vi "Begin.vi"(11 "Image Size":T1=enum."160x120") -> (0 "error out":errorcluster)   [LabVIEW 2012]
doc: "Called before other user functions, this VI is expected to open initial I/O refnums, load in file data, and do all program initialization. Notice that the <B>error out</B> terminal is simply used for data flow. Wiring it to other structures or subVIs ensures that this VI runs first."
uses:
  <vilib>/Rock Robotics/WPI/Camera/WPI_CameraImageSize.ctl
  <vilib>/Rock Robotics/WPI/Camera/WPI_CameraWhite Balance Values.ctl
  <vilib>/Rock Robotics/WPI/Camera/WPI_CameraExposure Values.ctl
  <vilib>/Rock Robotics/WPI/Camera/WPI_CameraFrameRate.ctl
  <vilib>/Rock Robotics/SystemInterfaces/DIO/FPGA_DIOPWMChannel.ctl
  <vilib>/Rock Robotics/WPI/Joystick/WPI_JoystickDeviceEnum.ctl
  <vilib>/Rock Robotics/SystemInterfaces/DIO/FPGA_DIOChannel.ctl
  <vilib>/Rock Robotics/WPI/Solenoid/WPI_SolenoidChannel.ctl
  <vilib>/Rock Robotics/SystemInterfaces/Typedef/FPGA_TypedefSolenoidModule.ctl
  <vilib>/Rock Robotics/SystemInterfaces/Typedef/FPGA_TypedefDigitalModule.ctl
  <vilib>/Rock Robotics/SystemInterfaces/DIO/FPGA_DIORelayChannel.ctl
  <vilib>/Rock Robotics/WPI/SafetyOutput/WPI_SafetyOutputConfigMenu.ctl
  <vilib>/Rock Robotics/WPI/MotorControl/WPI_MotorControlOpen Victor.vi
  <vilib>/Rock Robotics/WPI/Solenoid/WPI_SolenoidOpenSingle.vi
  <vilib>/Rock Robotics/WPI/MotorControl/WPI_MotorControlOpen Jaguar.vi
  Robot Global Data.vi
  <vilib>/Rock Robotics/WPI/RobotDrive/WPI_RobotDriveOpen4MotorWithJaguar.vi
  Autonomous Global Data.vi
  <vilib>/Rock Robotics/WPI/Compressor/WPI_CompressorGetSetRefNum.vi
  <vilib>/Rock Robotics/WPI/Encoder/WPI_EncoderType.ctl
  <vilib>/Rock Robotics/WPI/Counter/WPI_CounterDigitalInputToDigitalSource.vi
panel:
  out "1699-Autonomous.ini":string[][](array[string])=[["Autonomous Mode to run", "6"], ["Autonomous File No. to run (Mode 2 only)", "0"], ["Disance to Trave D1", "4.5"], ["Disance to Trave D2", "4.6"], ["Disance to Trave D3", "0"], ["Rate to tavel at R1", "-0.7"], ["Rate to tavel at R2", "-0.5"], ["Rate to tavel at R3", "0"], ["Key Shoot", "0"], ["Auto Type", "1"]]
  out "1699-preferences.ini":string[][](array[string])
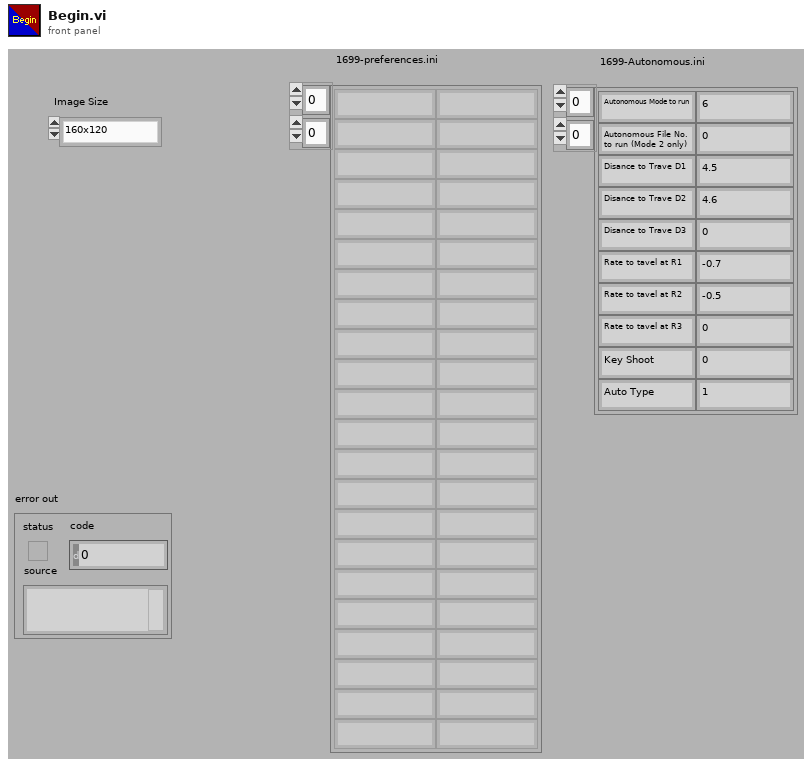
[diagram p1: front panel]
types:
  T1 = typedef "WPI_CameraImageSize.ctl" = enum16{"640x480", "320x240", "160x120"}
  T2 = typedef "WPI_SafetyOutputConfigMenu.ctl" = enum16{"Enable", "Disable"}
  T3 = typedef "FPGA_DIOChannel.ctl" = enum8{"DIO 1", "DIO 2", "DIO 3", "DIO 4", "DIO 5", "DIO 6", "DIO 7", "DIO 8", "DIO 9", "DIO 10", "DIO 11", "DIO 12", "DIO 13", "DIO 14", "Invalid"}
  T4 = typedef "FPGA_TypedefDigitalModule.ctl" = enum16{"Digital Module 1", "Digital Module 2"}
  T5 = typedef "FPGA_DIOPWMChannel.ctl" = enum8{"PWM 1", "PWM 2", "PWM 3", "PWM 4", "PWM 5", "PWM 6", "PWM 7", "PWM 8", "PWM 9", "PWM 10", "Invalid"}
  T6 = typedef "FPGA_DIORelayChannel.ctl" = enum8{"Relay 1", "Relay 2", "Relay 3", "Relay 4", "Relay 5", "Relay 6", "Relay 7", "Relay 8", "Invalid"}
  T7 = typedef "WPI_SolenoidChannel.ctl" = enum8{"Solenoid 1", "Solenoid 2", "Solenoid 3", "Solenoid 4", "Solenoid 5", "Solenoid 6", "Solenoid 7", "Solenoid 8", "Invalid"}
  T8 = typedef "FPGA_TypedefSolenoidModule.ctl" = enum16{"Solenoid Module 1", "Solenoid Module 2"}
  T9 = typedef "WPI_JoystickDeviceEnum.ctl" = enum16{"USB 1", "USB 2", "USB 3", "USB 4", "Kinect 1", "Kinect 2"}
  T10 = typedef "WPI_CameraFrameRate.ctl" = u32
  T11 = typedef "WPI_CameraExposure Values.ctl" = enum16{"Auto", "Flicker-free 50 Hz", "Flicker-free 60 Hz", "Hold current"}
  T12 = typedef "WPI_CameraWhite Balance Values.ctl" = enum16{"Auto", "Fixed indoor", "Fixed outdoor 1", "Fixed outdoor 2", "Fixed fluorescent 1", "Fixed fluorescent 2", "Hold current"}
  T13 = cluster{"[0]":dbl, "[1]":dbl, "[2]":dbl, "[3]":dbl, "[4]":dbl, "[5]":dbl, "[6]":dbl, "[7]":dbl, "[8]":dbl, "[9]":dbl, "[10]":dbl, "[11]":dbl, "[12]":dbl, "[13]":dbl, "[14]":dbl, "[15]":dbl, "[16]":dbl, "[17]":dbl, "[18]":dbl, "[19]":dbl}
  T14 = typedef "WPI_CameraDevRef.ctl" = cluster{"Camera Address":string, "CameraStatus":errorcluster, "Acquire Image Notifier":refnum<notifier>}
  T15 = typedef "WPI_RobotDriveDevRef.ctl" = cluster{"DevStatus":errorcluster, "Motors[]":T16[], "Square Inputs":bool, "Max Output":dbl, "Isochronous":bool}
  T16 = typedef "WPI_MotorControlDeviceRef.ctl" = cluster{"DeviceStatus":errorcluster, "Type":enum16{"PWM", "CAN"}, "PWM":cluster{"Digital Module":T4, "PWM Channel":T5, "DeadBand":T17}, "CAN":cluster{"Device Number":u8, "Control Mode":T18, "Semaphore":T19, "Max Vout":dbl}, "Invert":bool, "TransformRef":T20, "InvTransformRef":T20}
  T17 = typedef "WPI_PWMDeadband.ctl" = cluster{"Name":string, "maxPositivePwm":i32, "minPositivePwm":i32, "centerPwm":i32, "maxNegativePwm":i32, "minNegativePwm":i32, "angularRange":u16}
  T18 = typedef "WPI_CANJaguar_ControlMode.ctl" = enum8{"Percent VBus", "Current", "Speed", "Position", "Voltage"}
  T19 = typedef "Semaphore RefNum" = refnum<k1>
  T20 = typedef "WPI_PWMTransform_ConPane.ctl" = refnum<vi>
  T21 = typedef "WPI_EncoderType.ctl" = enum16{"1x", "2x", "4x"}
  T22 = typedef "WPI_DigitalInputDevRef.ctl" = cluster{"DevStatus":errorcluster, "DIO Channel":T3, "Digital Module":T4}
  T23 = typedef "FPGA_CounterEncoderSourceConvertionLVSourceType.ctl" = cluster{"DevStatus":errorcluster, "AnalogTriggerMode?":bool, "DigitalMode":cluster{"Digital Module":T4, "DIO Channel":T24}, "AnalogTriggerMode":cluster{"AnalogTriggerIndex":T25, "OutputType":T26}}
  T24 = typedef "FPGA_DIODigitalSourceChannel.ctl" = enum8{"DIO 1", "DIO 2", "DIO 3", "DIO 4", "DIO 5", "DIO 6", "DIO 7", "DIO 8", "DIO 9", "DIO 10", "DIO 11", "DIO 12", "DIO 13", "DIO 14", "Disabled"}
  T25 = typedef "FPGA_AnalogTriggerIndex.ctl" = enum8{"Trig 0", "Trig 1", "Trig 2", "Trig 3", "Trig 4", "Trig 5", "Trig 6", "Trig 7", "Invalid"}
  T26 = typedef "FPGA_AnalogTriggerOutType.ctl" = enum16{"InWindow", "TriggerState", "Rising", "Falling"}
  T27 = typedef "WPI_EncoderDevRef.ctl" = cluster{"DevStatus":errorcluster, "EncoderIndex":T28, "CounterIndex":T29, "DistancePerCount":dbl, "Decoding Type":T21}
  T28 = typedef "FPGA_EncoderIdx.ctl" = enum8{"Enc 0", "Enc 1", "Enc 2", "Enc 3", "Invalid"}
  T29 = typedef "FPGA_CounterCtrSystemIndex.ctl" = enum8{"Ctr 0", "Ctr 1", "Ctr 2", "Ctr 3", "Ctr 4", "Ctr 5", "Ctr 6", "Ctr 7", "Invalid"}
  T30 = typedef "WPI_JoystickDevRef.ctl" = cluster{"Device":T9}
  T31 = typedef "WPI_CompressorDevRef.ctl" = cluster{"DevStatus":errorcluster, "DigitalInputDevRef":T22, "RelayDevRef":T32}
  T32 = typedef "WPI_RelayDevRef.ctl" = cluster{"DevStatus":errorcluster, "Relay Channel":T6, "Digital Module":T4, "Relay Direction":T33}
  T33 = typedef "WPI_RelayDirection.ctl" = enum16{"Both directions", "Forward only", "Reverse only"}
  T34 = typedef "WPI_SolenoidDevRef.ctl" = cluster{"DevStatus":errorcluster, "Solenoid Module":T8, "Forward Solenoid Channel":T7, "Reverse Solenoid Channel":T7}
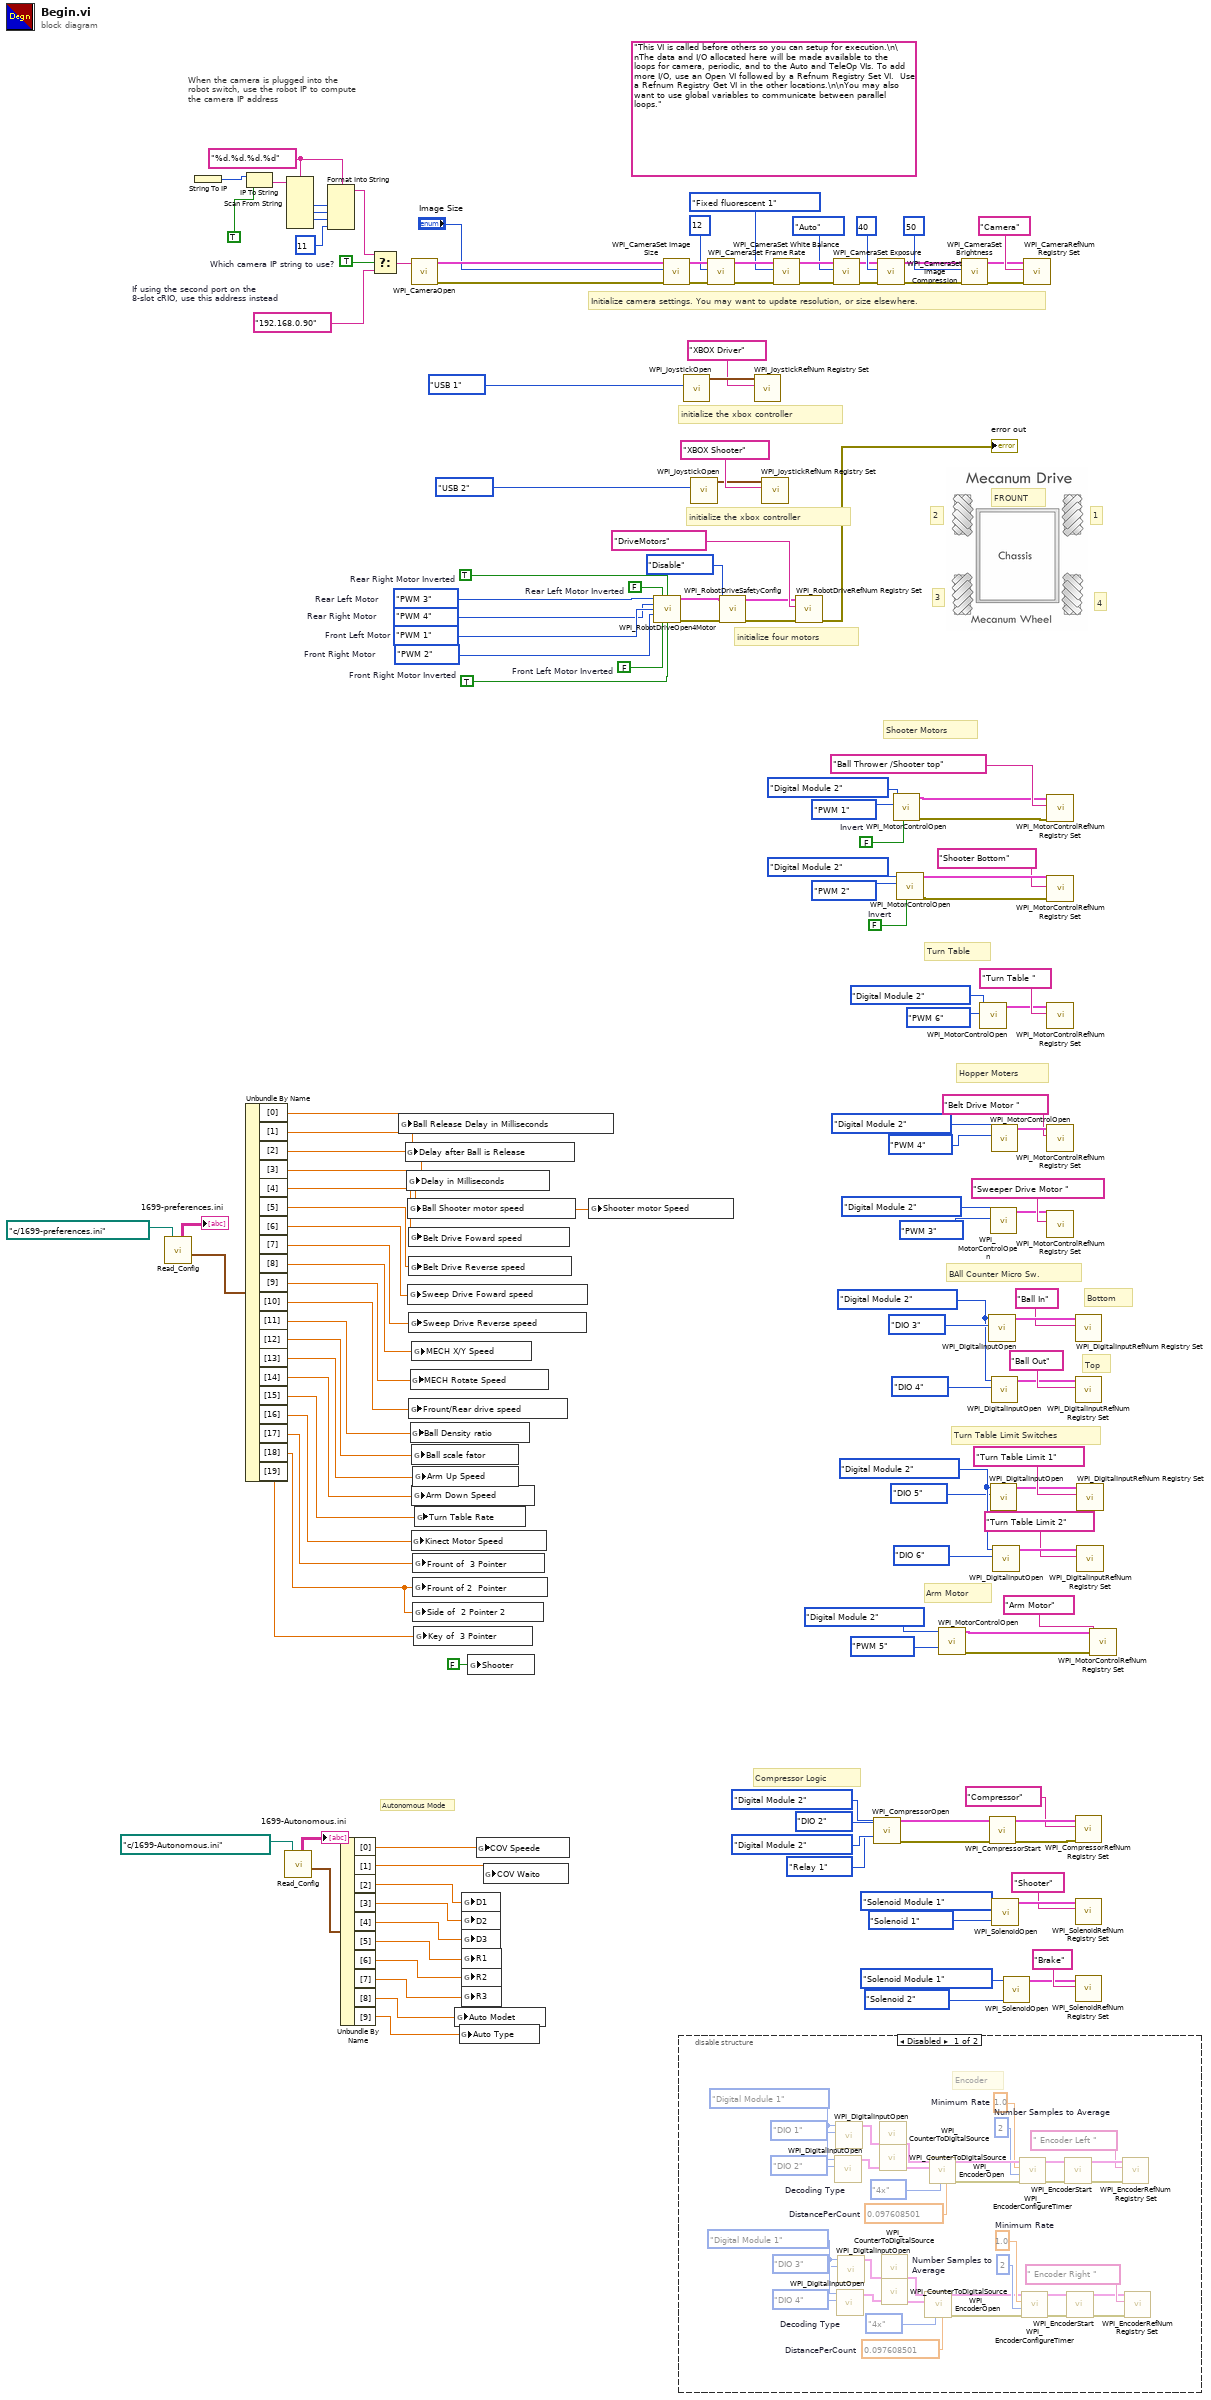
[diagram p0: block diagram]
diagram:
  w25 = FALSE  # Rear Left Motor Inverted
  w26 = FALSE  # Front Left Motor Inverted
  w36 = FPGA_TypedefDigitalModule."Digital Module 2" ("Digital Module (Module 1)")
  w43 = FALSE  # Invert
  w44 = FALSE  # Invert
  w94 = TRUE  # Front Right Motor Inverted
  w95 = TRUE  # Rear Right Motor Inverted
  w98 = FPGA_TypedefDigitalModule."Digital Module 2" ("Digital Module (Module 1)")
  w118 = FPGA_DIOPWMChannel."PWM 2"  # Front Right Motor
  w117 = FPGA_DIOPWMChannel."PWM 1"  # Front Left Motor
  w115 = FPGA_DIOPWMChannel."PWM 4"  # Rear Right Motor
  w114 = FPGA_DIOPWMChannel."PWM 3"  # Rear Left Motor
  w119 = TRUE  # Which camera IP string to use?
  w123 = "%d.%d.%d.%d" ("format string")
  (unwired) "This VI is called before others so you can setup for execution.\n\nThe data and I/O allocated here will be made available to the loops for camera, periodic, and to the Auto and TeleOp VIs. To add more I/O, use an Open VI followed by a Refnum Registry Set VI.  Use a Refnum Registry Get VI in the other locations.\n\nYou may also want to use global variables to communicate between parallel loops."
  w120 = "192.168.0.90"  # If using the second port on the 8-slot cRIO, use this address instead
  # "Autonomous Mode"
  # "FROUNT"
  # "Turn Table Limit Switches"
  # "Turn Table"
  # "Arm Motor"
  # "Top"
  # "Bottom"
  # "BAll Counter Micro Sw."
  # "Hopper Moters"
  # "Shooter Motors"
  # "Compressor Logic"
  # "initialize the xbox controller"
  # "1"
  # "4"
  # "3"
  # "2"
  # "initialize the xbox controller"
  # "initialize four motors"
  # "When the camera is plugged into the\nrobot switch, use the robot IP to compute\nthe camera IP address"
  # "Initialize camera settings. You may want to update resolution, or size elsewhere."
  n1 = call "Read_Config.vi"("configuration file path"=path "c:/1699-preferences.ini") -> ("PID Out"=w83:T13, "Array"=→"1699-preferences.ini":string[][])  [unwired: 2 in, 2 out]
  n2 = String To IP() -> (0:w130:u32)  [unwired: 1 in]
  n3 = Unbundle By Name(w83) -> ("[0]"=w93:dbl, "[1]"=w92:dbl, "[2]"=w91:dbl, "[3]"=w19:dbl, "[4]"=w90:dbl, "[5]"=w89:dbl, "[6]"=w88:dbl, "[7]"=w71:dbl, "[8]"=w70:dbl, "[9]"=w69:dbl, "[10]"=w68:dbl, "[11]"=w67:dbl, "[12]"=w66:dbl, "[13]"=w65:dbl, "[14]"=w64:dbl, "[15]"=w37:dbl, "[16]"=w29:dbl, "[17]"=w28:dbl, "[18]"=w20:dbl, "[19]"=w21:dbl)
  n4 = IP To String(1:TRUE ("dot notation? (F)"), 2:w130) -> (0:w128:string)
  n5 = call "Read_Config.vi"("configuration file path"=path "c:/1699-Autonomous.ini") -> ("PID Out"=w11:T13, "Array"=→"1699-Autonomous.ini":string[][])  [unwired: 2 in, 2 out]
  n6 = Scan From String(format string=w123, input string=w128) -> (output 1=w127:i32, output 2=w126:i32, output 3=w125:i32)  [unwired: 7 in, 3 out]
  n7 = Format Into String(format string=w123, w127, w126, w125, 11 ("Compression")) -> (resulting string=w121:string)  [unwired: 2 in, 1 out]
  n8 = Unbundle By Name(w11) -> ("[0]"=w10:dbl, "[1]"=w9:dbl, "[2]"=w8:dbl, "[3]"=w7:dbl, "[4]"=w6:dbl, "[5]"=w5:dbl, "[6]"=w4:dbl, "[7]"=w1:dbl, "[8]"=w3:dbl, "[9]"=w2:dbl)
  n9 = Select(t=w121, s=w119, f=w120) -> (s? t:f=w122:string)
  n10 = global write "Robot Global Data.vi" "Ball Release Delay in Milliseconds"(w93) -> ()
  n11 = global write "Robot Global Data.vi" "Delay after Ball is Release"(w92) -> ()
  n12 = global write "Robot Global Data.vi" "Delay in Milliseconds"(w91) -> ()
  n13 = global write "Robot Global Data.vi" "Ball Shooter motor speed"(w19) -> ()
  n14 = global write "Robot Global Data.vi" "Sweep Drive Foward speed"(w88) -> ()
  n15 = global write "Robot Global Data.vi" "Belt Drive Foward speed"(w90) -> ()
  n16 = global write "Robot Global Data.vi" "Belt Drive Reverse speed"(w89) -> ()
  n17 = global write "Robot Global Data.vi" "Sweep Drive Reverse speed"(w71) -> ()
  n18 = global write "Robot Global Data.vi" "Frount/Rear drive speed"(w68) -> ()
  n19 = global write "Robot Global Data.vi" "MECH Rotate Speed"(w69) -> ()
  n20 = global write "Robot Global Data.vi" "Ball Density ratio"(w67) -> ()
  n21 = call <vilib>:"WPI_CameraOpen.vi"("Camera Address"=w122) -> ("error out"=w142:errorcluster, "CameraDevRef"=w143:T14)  [unwired: 1 in, 8 out]
  n22 = global write "Robot Global Data.vi" "Kinect Motor Speed"(w29) -> ()
  n23 = global write "Robot Global Data.vi" "MECH X/Y Speed"(w70) -> ()
  n24 = global write "Robot Global Data.vi" "Ball scale fator"(w66) -> ()
  n25 = global write "Robot Global Data.vi" "Arm Down Speed"(w64) -> ()
  n26 = global write "Robot Global Data.vi" "Arm Up Speed"(w65) -> ()
  n27 = global write "Robot Global Data.vi" "Frount of  3 Pointer"(w28) -> ()
  n28 = global write "Robot Global Data.vi" "Frount of 2  Pointer"(w20) -> ()
  n29 = global write "Robot Global Data.vi" "Side of  2 Pointer 2"(w20) -> ()
  n30 = global write "Robot Global Data.vi" "Key of  3 Pointer"(w21) -> ()
  n31 = global write "Robot Global Data.vi" "Turn Table Rate"(w37) -> ()
  n32 = global write "Autonomous Global Data.vi" "Auto Modet"(w3) -> ()
  n33 = global write "Autonomous Global Data.vi" "Auto Type"(w2) -> ()
  n34 = global write "Autonomous Global Data.vi" "D1"(w8) -> ()
  n35 = global write "Autonomous Global Data.vi" "D2"(w7) -> ()
  n36 = global write "Autonomous Global Data.vi" "D3"(w6) -> ()
  n37 = global write "Autonomous Global Data.vi" "R1"(w5) -> ()
  n38 = global write "Autonomous Global Data.vi" "R2"(w4) -> ()
  n39 = global write "Autonomous Global Data.vi" "R3"(w1) -> ()
  n40 = global write "Robot Global Data.vi" "Shooter"(FALSE ("Shooter")) -> ()
  n41 = global write "Autonomous Global Data.vi" "COV Speede"(w10) -> ()
  n42 = global write "Autonomous Global Data.vi" "COV Waito"(w9) -> ()
  n43 = global write "Robot Global Data.vi" "Shooter motor Speed"(w19) -> ()
  n44 = call-poly <vilib>:"WPI_RobotDriveOpen4Motor.vi"("Rear Left Motor"=w114, "Rear Left Motor Inverted"=w25, "Rear Right Motor Inverted"=w95, "Rear Right Motor"=w115, "Front Left Motor"=w117, "Front Right Motor"=w118, "Front Left Motor Inverted"=w26, "Front Right Motor Inverted"=w94) -> ("RobotDriveDevRef"=w18:T15, "error out"=w15:errorcluster)  [unwired: 1 in, 5 out]
  n45 = call <vilib>:"WPI_CameraSet Image Size.vi"("error in (no error)"=w142, "Image Size"="Image Size", "CameraDevRef"=w143) -> ("error out"=w141:errorcluster, "CameraDevRef Out"=w144:T14)  [unwired: 7 out]
  n46 = disable-structure shown="Disabled" {
    frame Disabled {
      w169 = FPGA_TypedefDigitalModule."Digital Module 1" ("Digital Module (Module 1)")
      w162 = 0.097608501  # DistancePerCount
      w161 = WPI_EncoderType."4x"  # Decoding Type
      w160 = u8 2  # Number Samples to Average
      w159 = 1.0  # Minimum Rate
      w170 = FPGA_TypedefDigitalModule."Digital Module 1" ("Digital Module (Module 1)")
      w177 = 0.097608501  # DistancePerCount
      w178 = WPI_EncoderType."4x"  # Decoding Type
      w179 = u8 2  # Number Samples to Average
      w180 = 1.0  # Minimum Rate
      # "Encoder"
      n47 = call <vilib>:"WPI_DigitalInputOpen.vi"("DIO Channel"=FPGA_DIOChannel."DIO 2", "Digital Module (Module 1)"=w170) -> ("DigitalInputDevRef"=w174:T22)  [unwired: 8 in, 1 out]
      n48 = call <vilib>:"WPI_DigitalInputOpen.vi"("DIO Channel"=FPGA_DIOChannel."DIO 1", "Digital Module (Module 1)"=w170) -> ("DigitalInputDevRef"=w173:T22)  [unwired: 8 in, 1 out]
      n49 = call <vilib>:"WPI_DigitalInputOpen.vi"("DIO Channel"=FPGA_DIOChannel."DIO 4", "Digital Module (Module 1)"=w169) -> ("DigitalInputDevRef"=w165:T22)  [unwired: 8 in, 1 out]
      n50 = call <vilib>:"WPI_DigitalInputOpen.vi"("DIO Channel"=FPGA_DIOChannel."DIO 3", "Digital Module (Module 1)"=w169) -> ("DigitalInputDevRef"=w166:T22)  [unwired: 8 in, 1 out]
      n51 = call-poly <vilib>:"WPI_CounterToDigitalSource.vi"("DigitalInputDevRef"=w173) -> ("Digital Source"=w175:T23)  [unwired: 6 in]
      n52 = call-poly <vilib>:"WPI_CounterToDigitalSource.vi"("DigitalInputDevRef"=w174) -> ("Digital Source"=w176:T23)  [unwired: 6 in]
      n53 = call-poly <vilib>:"WPI_CounterToDigitalSource.vi"("DigitalInputDevRef"=w166) -> ("Digital Source"=w164:T23)  [unwired: 6 in]
      n54 = call-poly <vilib>:"WPI_CounterToDigitalSource.vi"("DigitalInputDevRef"=w165) -> ("Digital Source"=w163:T23)  [unwired: 6 in]
      n55 = call <vilib>:"WPI_EncoderOpen.vi"("DistancePerCount"=w162, "Decoding Type"=w161, "BSource"=w163, "ASource"=w164) -> ("error out"=w158:errorcluster, "EncoderDevRef"=w152:T27)  [unwired: 6 in]
      n56 = call <vilib>:"WPI_EncoderOpen.vi"("DistancePerCount"=w177, "Decoding Type"=w178, "BSource"=w176, "ASource"=w175) -> ("error out"=w181:errorcluster, "EncoderDevRef"=w187:T27)  [unwired: 6 in]
      n57 = call <vilib>:"WPI_EncoderConfigureTimer.vi"("error in (no error)"=w181, "Number Samples to Average"=w179, "Minimum Rate"=w180, "EncoderDevRef"=w187) -> ("error out"=w182:errorcluster, "EncoderDevRef"=w186:T27)  [unwired: 6 in]
      n58 = call <vilib>:"WPI_EncoderConfigureTimer.vi"("error in (no error)"=w158, "Number Samples to Average"=w160, "Minimum Rate"=w159, "EncoderDevRef"=w152) -> ("error out"=w157:errorcluster, "EncoderDevRef"=w153:T27)  [unwired: 6 in]
      n59 = call <vilib>:"WPI_EncoderStart.vi"("error in (no error)"=w182, "EncoderDevRef"=w186) -> ("error out"=w183:errorcluster, "EncoderDevRef"=w185:T27)  [unwired: 8 in]
      n60 = call <vilib>:"WPI_EncoderStart.vi"("error in (no error)"=w157, "EncoderDevRef"=w153) -> ("error out"=w156:errorcluster, "EncoderDevRef"=w154:T27)  [unwired: 8 in]
      n61 = call <vilib>:"WPI_EncoderRefNum Registry Set.vi"("error in (no error)"=w183, "refnum name"=" Encoder Left ", "EncoderDevRef"=w185) -> ()  [unwired: 7 in, 2 out]
      n62 = call <vilib>:"WPI_EncoderRefNum Registry Set.vi"("error in (no error)"=w156, "refnum name"=" Encoder Right ", "EncoderDevRef"=w154) -> ()  [unwired: 7 in, 2 out]
    }
    frame Enabled {
    }
  }
  n63 = call <vilib>:"WPI_JoystickOpen.vi"("JoystickDevice"=WPI_JoystickDeviceEnum."USB 1") -> ("JoystickDevRef"=w82:T30)  [unwired: 10 out]
  n64 = call <vilib>:"WPI_JoystickOpen.vi"("JoystickDevice"=WPI_JoystickDeviceEnum."USB 2") -> ("JoystickDevRef"=w112:T30)  [unwired: 10 out]
  n65 = call <vilib>:"WPI_CameraSet Frame Rate.vi"("error in (no error)"=w141, "Frame Rate (fps)"=T10 12, "CameraDevRef"=w144) -> ("error out"=w140:errorcluster, "CameraDevRef Out"=w146:T14)  [unwired: 7 out]
  n66 = call <vilib>:"WPI_RobotDriveSafetyConfig.vi"("error in (no error)"=w15, "mode"=WPI_SafetyOutputConfigMenu."Disable", "RobotDriveDevRef"=w18) -> ("error out"=w16:errorcluster, "RobotDriveDevRef"=w17:T15)  [unwired: 7 in]
  n67 = call <vilib>:"WPI_JoystickRefNum Registry Set.vi"("refnum name"="XBOX Driver", "JoystickDevRef"=w82) -> ()  [unwired: 1 in, 9 out]
  n68 = call <vilib>:"WPI_JoystickRefNum Registry Set.vi"("refnum name"="XBOX Shooter", "JoystickDevRef"=w112) -> ()  [unwired: 1 in, 9 out]
  n69 = call <vilib>:"WPI_CameraSet White Balance.vi"("error in (no error)"=w140, "White Balance"=WPI_CameraWhite_Balance_Values."Fixed fluorescent 1", "CameraDevRef"=w146) -> ("error out"=w139:errorcluster, "CameraDevRef Out"=w145:T14)  [unwired: 7 out]
  n70 = call <vilib>:"WPI_RobotDriveRefNum Registry Set.vi"("error in (no error)"=w16, "refnum name"="DriveMotors", "RobotDriveDevRef"=w17) -> ("error out"=→"error out":errorcluster)  [unwired: 8 out]
  n71 = call <vilib>:"WPI_CameraSet Exposure.vi"("error in (no error)"=w139, "Exposure"=WPI_CameraExposure_Values."Auto", "CameraDevRef"=w145) -> ("error out"=w138:errorcluster, "CameraDevRef Out"=w148:T14)  [unwired: 7 out]
  n72 = call <vilib>:"WPI_CompressorOpen.vi"("Pressure Switch Digital Module (Module 1)"=FPGA_TypedefDigitalModule."Digital Module 2", "Pressure Switch DIO Channel"=FPGA_DIOChannel."DIO 2", "Relay Digital Module (Module 1)"=FPGA_TypedefDigitalModule."Digital Module 2", "Relay Channel"=FPGA_DIORelayChannel."Relay 1") -> ("CompressorDevRef"=w63:T31, "error out"=w62:errorcluster)  [unwired: 10 in]
  n73 = call <vilib>:"WPI_CameraSet Image Compression.vi"("error in (no error)"=w138, "Compression"=40, "CameraDevRef"=w148) -> ("error out"=w137:errorcluster, "CameraDevRef Out"=w147:T14)  [unwired: 7 out]
  n74 = call-poly <vilib>:"WPI_MotorControlOpen.vi"("Invert"=w44, "PWM Channel"=FPGA_DIOPWMChannel."PWM 1", "Digital Module (Module 1)"=FPGA_TypedefDigitalModule."Digital Module 2") -> ("error out"=w51:errorcluster, "MotorControlDeviceRef"=w52:T16)  [unwired: 7 in]
  n75 = call-poly <vilib>:"WPI_MotorControlOpen.vi"("Invert"=w43, "PWM Channel"=FPGA_DIOPWMChannel."PWM 2", "Digital Module (Module 1)"=FPGA_TypedefDigitalModule."Digital Module 2") -> ("error out"=w49:errorcluster, "MotorControlDeviceRef"=w50:T16)  [unwired: 7 in]
  n76 = call-poly <vilib>:"WPI_MotorControlOpen.vi"("PWM Channel"=FPGA_DIOPWMChannel."PWM 5", "Digital Module (Module 1)"=FPGA_TypedefDigitalModule."Digital Module 2") -> ("error out"=w22:errorcluster, "MotorControlDeviceRef"=w23:T16)  [unwired: 8 in]
  n77 = call <vilib>:"WPI_CameraSet Brightness.vi"("error in (no error)"=w137, "Brightness"=50, "CameraDevRef"=w147) -> ("error out"=w135:errorcluster, "CameraDevRef Out"=w136:T14)  [unwired: 7 out]
  n78 = call-poly <vilib>:"WPI_MotorControlOpen.vi"("PWM Channel"=FPGA_DIOPWMChannel."PWM 6", "Digital Module (Module 1)"=FPGA_TypedefDigitalModule."Digital Module 2") -> ("MotorControlDeviceRef"=w39:T16)  [unwired: 8 in, 1 out]
  n79 = call <vilib>:"WPI_DigitalInputOpen.vi"("DIO Channel"=FPGA_DIOChannel."DIO 3", "Digital Module (Module 1)"=w98) -> ("DigitalInputDevRef"=w104:T22)  [unwired: 8 in, 1 out]
  n80 = call <vilib>:"WPI_CompressorStart.vi"("error in (no error)"=w62, "CompressorDevRef"=w63) -> ("error out"=w61:errorcluster, "CompressorDevRef"=w60:T31)  [unwired: 8 in]
  n81 = call-poly <vilib>:"WPI_MotorControlOpen.vi"("PWM Channel"=FPGA_DIOPWMChannel."PWM 3", "Digital Module (Module 1)"=FPGA_TypedefDigitalModule."Digital Module 2") -> ("MotorControlDeviceRef"=w105:T16)  [unwired: 8 in, 1 out]
  n82 = call <vilib>:"WPI_DigitalInputOpen.vi"("DIO Channel"=FPGA_DIOChannel."DIO 5", "Digital Module (Module 1)"=w36) -> ("DigitalInputDevRef"=w31:T22)  [unwired: 8 in, 1 out]
  n83 = call-poly <vilib>:"WPI_MotorControlOpen.vi"("PWM Channel"=FPGA_DIOPWMChannel."PWM 4", "Digital Module (Module 1)"=FPGA_TypedefDigitalModule."Digital Module 2") -> ("MotorControlDeviceRef"=w108:T16)  [unwired: 8 in, 1 out]
  n84 = call <vilib>:"WPI_DigitalInputOpen.vi"("DIO Channel"=FPGA_DIOChannel."DIO 4", "Digital Module (Module 1)"=w98) -> ("DigitalInputDevRef"=w99:T22)  [unwired: 8 in, 1 out]
  n85 = call-poly <vilib>:"WPI_SolenoidOpen.vi"("Solenoid Channel"=WPI_SolenoidChannel."Solenoid 1", "Solenoid Module (Module 1)"=FPGA_TypedefSolenoidModule."Solenoid Module 1") -> ("SolenoidDevRef"=w79:T34)  [unwired: 8 in, 1 out]
  n86 = call <vilib>:"WPI_DigitalInputOpen.vi"("DIO Channel"=FPGA_DIOChannel."DIO 6", "Digital Module (Module 1)"=w36) -> ("DigitalInputDevRef"=w35:T22)  [unwired: 8 in, 1 out]
  n87 = call-poly <vilib>:"WPI_SolenoidOpen.vi"("Solenoid Channel"=WPI_SolenoidChannel."Solenoid 2", "Solenoid Module (Module 1)"=FPGA_TypedefSolenoidModule."Solenoid Module 1") -> ("SolenoidDevRef"=w72:T34)  [unwired: 8 in, 1 out]
  n88 = call <vilib>:"WPI_CameraRefNum Registry Set.vi"("error in (no error)"=w135, "refnum name"="Camera", "CameraDevRef"=w136) -> ()  [unwired: 9 out]
  n89 = call <vilib>:"WPI_MotorControlRefNum Registry Set.vi"("error in (no error)"=w51, "refnum name"="Ball Thrower /Shooter top", "MotorControlDevRef"=w52) -> ()  [unwired: 7 in, 2 out]
  n90 = call <vilib>:"WPI_MotorControlRefNum Registry Set.vi"("error in (no error)"=w49, "refnum name"="Shooter Bottom", "MotorControlDevRef"=w50) -> ()  [unwired: 7 in, 2 out]
  n91 = call <vilib>:"WPI_MotorControlRefNum Registry Set.vi"("refnum name"="Turn Table ", "MotorControlDevRef"=w39) -> ()  [unwired: 8 in, 2 out]
  n92 = call <vilib>:"WPI_MotorControlRefNum Registry Set.vi"("refnum name"="Belt Drive Motor ", "MotorControlDevRef"=w108) -> ()  [unwired: 8 in, 2 out]
  n93 = call <vilib>:"WPI_MotorControlRefNum Registry Set.vi"("refnum name"="Sweeper Drive Motor ", "MotorControlDevRef"=w105) -> ()  [unwired: 8 in, 2 out]
  n94 = call <vilib>:"WPI_DigitalInputRefNum Registry Set.vi"("refnum name"="Ball In", "DigitalInputDevRef"=w104) -> ()  [unwired: 8 in, 2 out]
  n95 = call <vilib>:"WPI_DigitalInputRefNum Registry Set.vi"("refnum name"="Ball Out", "DigitalInputDevRef"=w99) -> ()  [unwired: 8 in, 2 out]
  n96 = call <vilib>:"WPI_CompressorRefNum Registry Set.vi"("error in (no error)"=w61, "refnum name"="Compressor", "CompressorDevRef"=w60) -> ()  [unwired: 7 in, 2 out]
  n97 = call <vilib>:"WPI_SolenoidRefNum Registry Set.vi"("refnum name"="Shooter", "SolenoidDevRef"=w79) -> ()  [unwired: 8 in, 2 out]
  n98 = call <vilib>:"WPI_SolenoidRefNum Registry Set.vi"("refnum name"="Brake", "SolenoidDevRef"=w72) -> ()  [unwired: 8 in, 2 out]
  n99 = call <vilib>:"WPI_DigitalInputRefNum Registry Set.vi"("refnum name"="Turn Table Limit 1", "DigitalInputDevRef"=w31) -> ()  [unwired: 8 in, 2 out]
  n100 = call <vilib>:"WPI_DigitalInputRefNum Registry Set.vi"("refnum name"="Turn Table Limit 2", "DigitalInputDevRef"=w35) -> ()  [unwired: 8 in, 2 out]
  n101 = call <vilib>:"WPI_MotorControlRefNum Registry Set.vi"("error in (no error)"=w22, "refnum name"="Arm Motor", "MotorControlDevRef"=w23) -> ()  [unwired: 7 in, 2 out]
